vi "DAQ Interface.vi"() -> ()   [LabVIEW 2021]
uses:
  <vilib>/DAQmx/read.llb/DAQmx Read (Analog 1D DBL 1Chan NSamp).vi
  <vilib>/DAQmx/create/channels.llb/DAQmx Create Channel (AI-Voltage-Basic).vi
  <vilib>/DAQmx/configure/timing.llb/DAQmx Timing (Sample Clock).vi
  <vilib>/DAQmx/miscellaneous.llb/DAQmx Fill In Error Info.vi
  <resource>/objmgr/daqmx.rc
panel:
  in  "minimum value":dbl=-5.0 format="%0.2f"
  in  "maximum value":dbl=5.0 format="%0.2f"
  in  "physical channels":tag="Dev1/ai7"
  in  "Update params":bool
  in  "source":tag="OnboardClock"
  in  "rate":dbl=250000.0
  in  "number of samples":i32=10000
  out "Waveform Chart":dbl(graph)
  in  "stop":bool
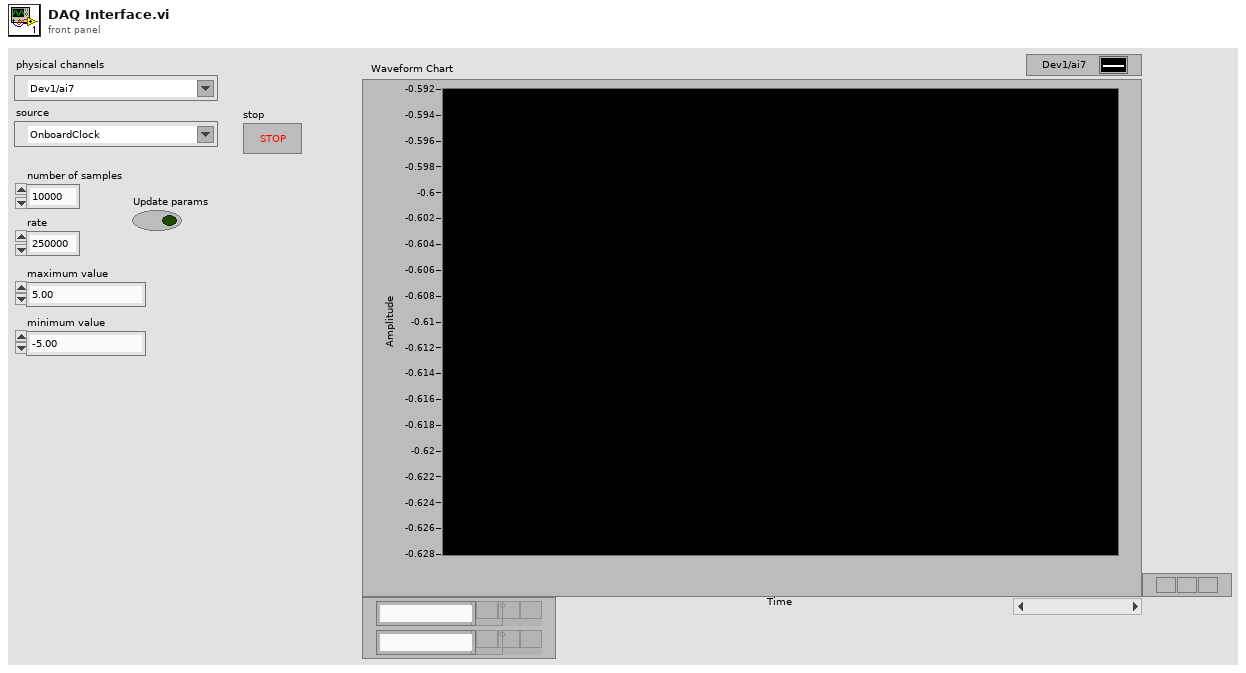
[diagram p1: front panel]
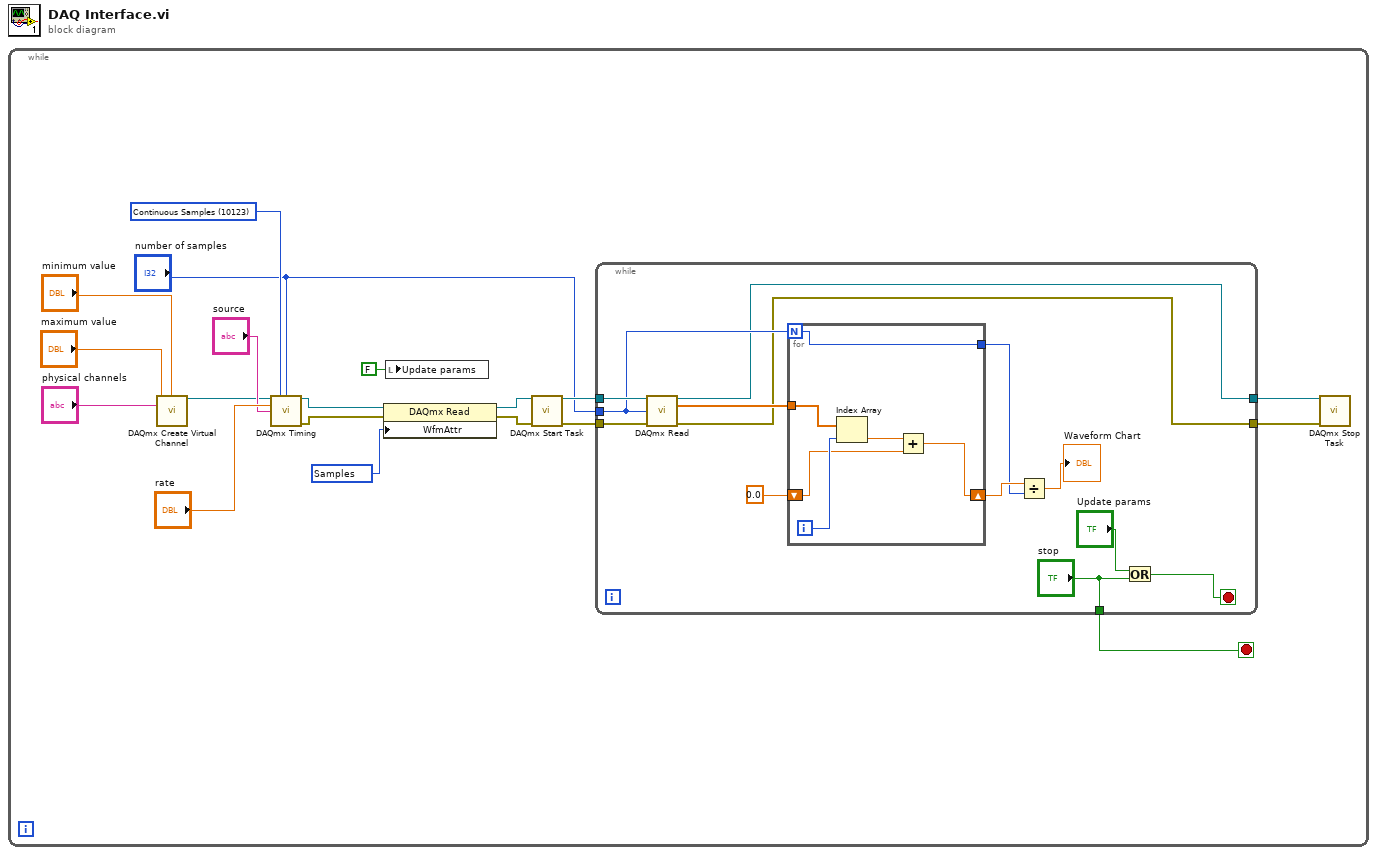
[diagram p0: block diagram]
diagram:
  n1 = while {
    stop <- w7 stop-if-true
    w12 = 10287 items=["Samples"=10287, "Samples and Timing"=10140, "Samples, Timing, and Attributes"=10141] ("WfmAttr")
    w15 = 10123 items=["Finite Samples"=10178, "Continuous Samples"=10123, "Hardware Timed Single Point"=12522] ("sample mode")
    n2 = call-poly <vilib>:"DAQmx Create Virtual Channel.vi"("maximum value"="maximum value", "minimum value"="minimum value", "physical channels"="physical channels") -> ("task out"=w13:refnum<k21>)  [unwired: 11 in, 1 out]
    n3 = call-poly <vilib>:"DAQmx Timing.vi"("task/channels in"=w13, "sample mode"=w15, "samples per channel"="number of samples", "rate"="rate", "source"="source") -> ("task out"=w11:refnum<k21>, "error out"=w9:errorcluster)  [unwired: 9 in]
    n4 = property class="DAQmx Read"(reference=w11, error in=w9, "WfmAttr"=w12) -> (reference out=w10:refnum<k21>, error out=w8:errorcluster)
    n5 = local write "Update params"(FALSE ("Update params")) -> ()
    n6 = call <vilib>:"DAQmx Start Task.vi"("task/channels in"=w10, "error in"=w8) -> ("task out"=w18:refnum<k21>, "error out"=w17:errorcluster)  [unwired: 12 in]
    n7 = while {
      tunnel: [w21] -> w5
      tunnel: [w20] -> w4
      tunnel: w18 -> [w32]
      tunnel: w17 -> [w31]
      tunnel: "number of samples" -> [w26]
      tunnel: ["stop"] -> w7
      stop <- w23 stop-if-true
      n8 = call-poly <vilib>:"DAQmx Read.vi"("task/channels in"=w32, "number of samples per channel"=w26, "error in"=w31) -> ("task out"=w21:refnum<k21>, "data"=w30:dbl[], "error out"=w20:errorcluster)  [unwired: 10 in]
      n9 = for {
        N: w26 -> [w33]
        shift-right: [w34] -> w28
        shift-left: 0.0 -> [w35]
        tunnel: w30 -> [w37]
        tunnel: [w33] -> w27
        i -> [w38]
        n10 = Index Array(array=w37, index=w38) -> (element=w36:dbl)
        n11 = Add(x=w36, y=w35) -> (x+y=w34:dbl)
      }
      n12 = Divide(x=w28, y=w27) -> (x/y=→"Waveform Chart":dbl)
      n13 = Or(x="Update params", y="stop") -> (x .or. y?=w23:bool)
    }
    n14 = call <vilib>:"DAQmx Stop Task.vi"("task/channels in"=w5, "error in"=w4) -> ()  [unwired: 12 in, 2 out]
  }
